vi "DataLoggingSessionStateChange Event Callback.vi"(4 "State Change Event":refnum<user-event>, 5 "Event Data":cluster{"sender":refnum<k24>, "e":refnum<k24>}, 6 "Data Logging Manager Ref":T1, 7 "Event Common Data":T2) -> ()   [LabVIEW 2020, in "NI_VS Data Logging API.lvlib"]
uses:
  <vilib>/NI VeriStand/Execution/DataLogging/NI_VS Data Logging API.lvlib
  <vilib>/NI VeriStand/Execution/DataLogging/IDataLogging Ref.ctl
  NationalInstruments.VeriStand.ClientAPI
  <vilib>/NI VeriStand/Execution/DataLogging/Data Logging Session State Change Event Data.ctl
  <vilib>/NI VeriStand/Execution/DataLogging/Data Logging Session State.ctl
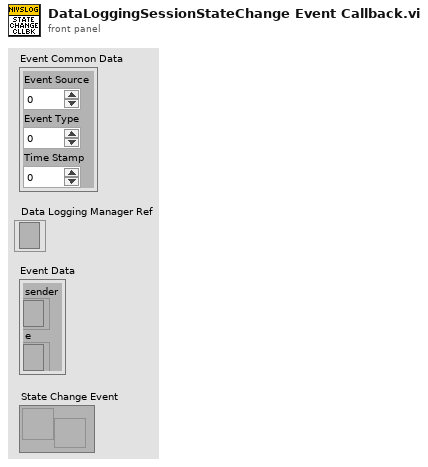
[diagram p1: front panel]
types:
  T1 = typedef "NI_VS Data Logging API.lvlib/IDataLogging Ref.ctl" = refnum<k24>
  T2 = cluster{"Event Source":i32, "Event Type":u32, "Time Stamp":u32}
  T3 = typedef "NI_VS Data Logging API.lvlib/Data Logging Session State Change Event Data.ctl" = cluster{"Session Name":string, "Session State":T4}
  T4 = typedef "NI_VS Data Logging API.lvlib/Data Logging Session State.ctl" = enum16{"Waiting on Trigger", "Triggered", "Post-Trigger", "Complete", "Idle", "Error"}
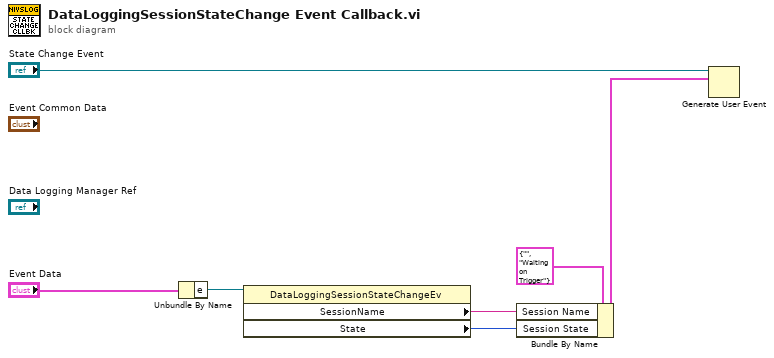
[diagram p0: block diagram]
diagram:
  n1 = Unbundle By Name("Event Data") -> ("e"=w3:refnum<k24>)
  n2 = property class="DataLoggingSessionStateChangeEv"(reference=w3) -> ("SessionName"=w2:string, "State"=w1:i32)  [unwired: 1 in, 2 out]
  n3 = Bundle By Name(cluster=T3 {"Session Name"="", "Session State"=enum."Waiting on Trigger"} ("event data"), "Session Name"=w2, "Session State"=w1) -> (w5:T3)
  n4 = Generate User Event(user event="State Change Event", event data cluster=w5) -> ()  [unwired: 2 in, 2 out]
